vi "Python String to LabVIEW Data (Boolean).vi"(8 "error in (no error)":errorcluster, 9 "type":bool, 10 "Python String":string) -> (0 "error out":errorcluster, 2 "LabVIEW Data":bool)   [LabVIEW 2020, in "jki_python_data_tools.lvlib"]
doc: "Reads a value associated with key in a specified section of the configuration data identified by refnum. If \"key\" input is not specified, the name of the variant object is used as the key. the \"found?\" output will be TRUE for compount objects (clusters) only if all elements (recursively) are found.\n\nFor example a Boolean named \"Enable\" with a value of TRUE would correspond to the key-value pair:\n\nEnable=TRUE"
uses:
  jki_python_data_tools.lvlib
panel:
  # "Copyright © 2003-2009 JKI. All rights reserved.\n\nAuthor:\nPhilippe Guerit [philippe.guerit@jameskring.com]\nJim Kring [jim.kring@jameskring.com]\n\nThis library is provided \"AS IS\" ,WITHOUT WARRANTIES OR \nCONDITIONS OF ANY KIND, either express or implied.\n\nJames Kring, Inc. -- http://www.jameskring.com"
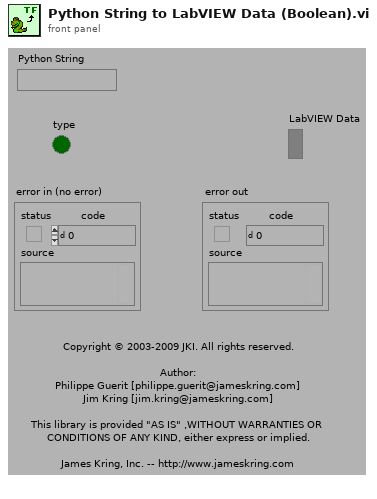
[diagram p1: front panel]
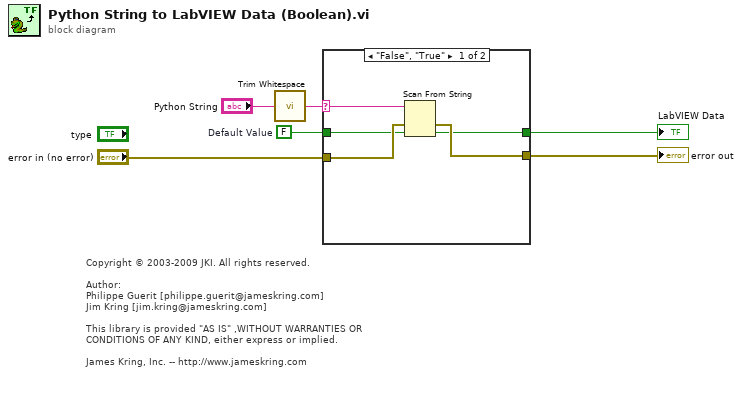
[diagram p0: block diagram]
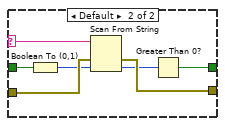
[diagram p2: hidden frame]
diagram:
  w6 = FALSE  # Default Value
  # "Copyright © 2003-2009 JKI. All rights reserved.\n\nAuthor:\nPhilippe Guerit [philippe.guerit@jameskring.com]\nJim Kring [jim.kring@jameskring.com]\n\nThis library is provided \"AS IS\" ,WITHOUT WARRANTIES OR \nCONDITIONS OF ANY KIND, either express or implied.\n\nJames Kring, Inc. -- http://www.jameskring.com"
  n1 = call <vilib>:"Trim Whitespace.vi"("string"="Python String") -> ("trimmed string"=w1:string)  [unwired: 1 in]
  n2 = case shown="\"False\", \"True\"" w1 {
    selector: w1 -> [w7 w12]
    tunnel: w6 -> [w9 w18]
    tunnel: "error in (no error)" -> [w11 w17]
    tunnel: [w10 w16] -> w5
    tunnel: [w8 w13] -> w4
    frame "False", "True" {
      n3 = Scan From String(input string=w7, error in=w11, default 1=w9) -> (error out=w10:errorcluster, output 1=w8:bool)  [unwired: 2 in, 2 out]
    }
    frame Default {
      n4 = Boolean To (0,1)(Boolean=w18) -> (0, 1=w15:i16)
      n5 = Scan From String(input string=w12, error in=w17, default 1=w15) -> (error out=w16:errorcluster, output 1=w14:i16)  [unwired: 2 in, 2 out]
      n6 = Greater Than 0?(x=w14) -> (x > 0?=w13:bool)
    }
  }
  "error out" <- w5
  "LabVIEW Data" <- w4
